vi "Main.vi"(8 "error in (no error)":errorcluster, 11 "Trace in":refnum<class "Trace.lvclass">) -> (0 "error out":errorcluster, 3 "Trace out":refnum<class "Trace.lvclass">)   [LabVIEW 2012, in "Trace.lvclass"]
doc: "Main VI of the component. This should contain the GUI of your component and be called when creating an executable."
uses:
  Trace.lvclass
  <vilib>/Distrio/Murmex/Murmex/Murmex.lvclass
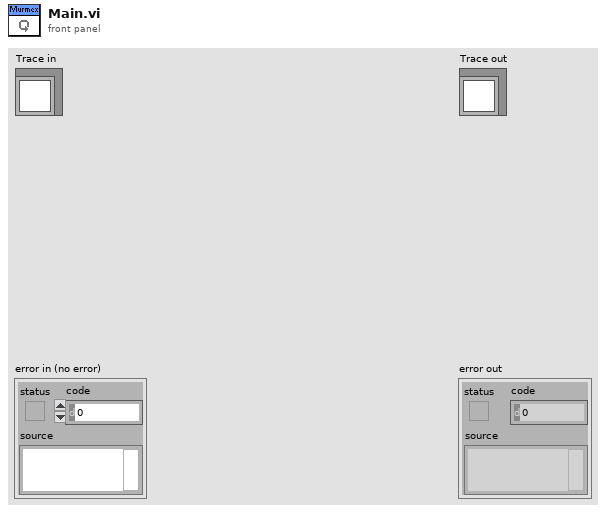
[diagram p1: front panel]
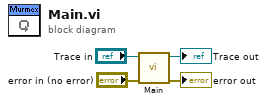
[diagram p0: block diagram]
diagram:
  n1 = call-parent "Main.vi"("error in (no error)"="error in (no error)", "Murmex in"="Trace in") -> ("error out"=→"error out":errorcluster, "Murmex out"=→"Trace out":refnum<class "Trace.lvclass">)  [unwired: 8 in]
